vi "BPtrayCalib.vi"(0 "Operation":enum16{"Manual", "Automatic"}(ring)=enum."Automatic", 1 "Zone":enum16{"ZoneA", "ZoneB", "ZoneC", "ZoneD"}(ring), 2 "Autofocus":T4={"Enable"=TRUE, "InitialStepSize"=0.05, "Tolerance"=0.02, "Abort"=FALSE} {"Tolerance" format="%#_13g"}, 7 "StopJoyStick":bool, 9 "VisibilityInCamera":enum16{"JoyStick", "AllVisible"}(ring)=enum."AllVisible", 11 "error in (no error)":errorcluster, 13 "SaveImagesLog":bool=TRUE) -> (6 "Image":T5(plugin-control), 8 "Image 2":T5[](array[plugin-control]) caption="AllImages", 15 "error out":errorcluster)   [LabVIEW 2021]
uses:
  <vilib>/userDefined/High Color/IMAQdx.ctl
  <vilib>/Analysis/coordinate.llb/2D Cartesian Coordinate Rotation (Scalar).vi
  include/GlobalVariables.vi
  Other Models/2010/Motion/AbortSingle.vi
  <vilib>/Analysis/NI_AALPro.lvlib
  <vilib>/vision/driver/NI_Vision_Acquisition_Software.lvlib
panel:
  out "CameraGcode2":string
  out "AllMatches":T1(array[cluster]) {"Bounding Box"."y" format="%.2f"; "Bounding Box"."x" format="%.2f"; "Score" format="%.2f"; "Scale" format="%.2f"; "Angle" format="%.2f"; "Position"."y" format="%.2f"; "Position"."x" format="%.2f"}
  in  "MatchParameters":T2={"Number of Matches Requested"=1, "Minimum Match Score"=500.0, "Angle Ranges"=[{"Start Angle"=0.0, "End Angle"=0.0}]}
  out "OutputFile2":string
  out "XYZU_Back":string
  out "XYZU_Front":string
  out "TrayAngle":dbl
  in  "TrayID":string="1"
  in  "Camera":T3="cam1"
  out "OutputFile1":string
  out "spreadsheet string 2":string
  out "spreadsheet string":string
  in  "ModuleName":string="T1"
  out "SyringeY":dbl format="%#_7g"
  out "SyringeX":dbl format="%#_7g"
  in  "CamToSyringeYoffset":dbl=126.651
  in  "CamToSyringeXoffset":dbl=167.702
  out "FileUsedForFiducials":string
  out "UsedCoordinates":string
  out "CameraGcode1":string
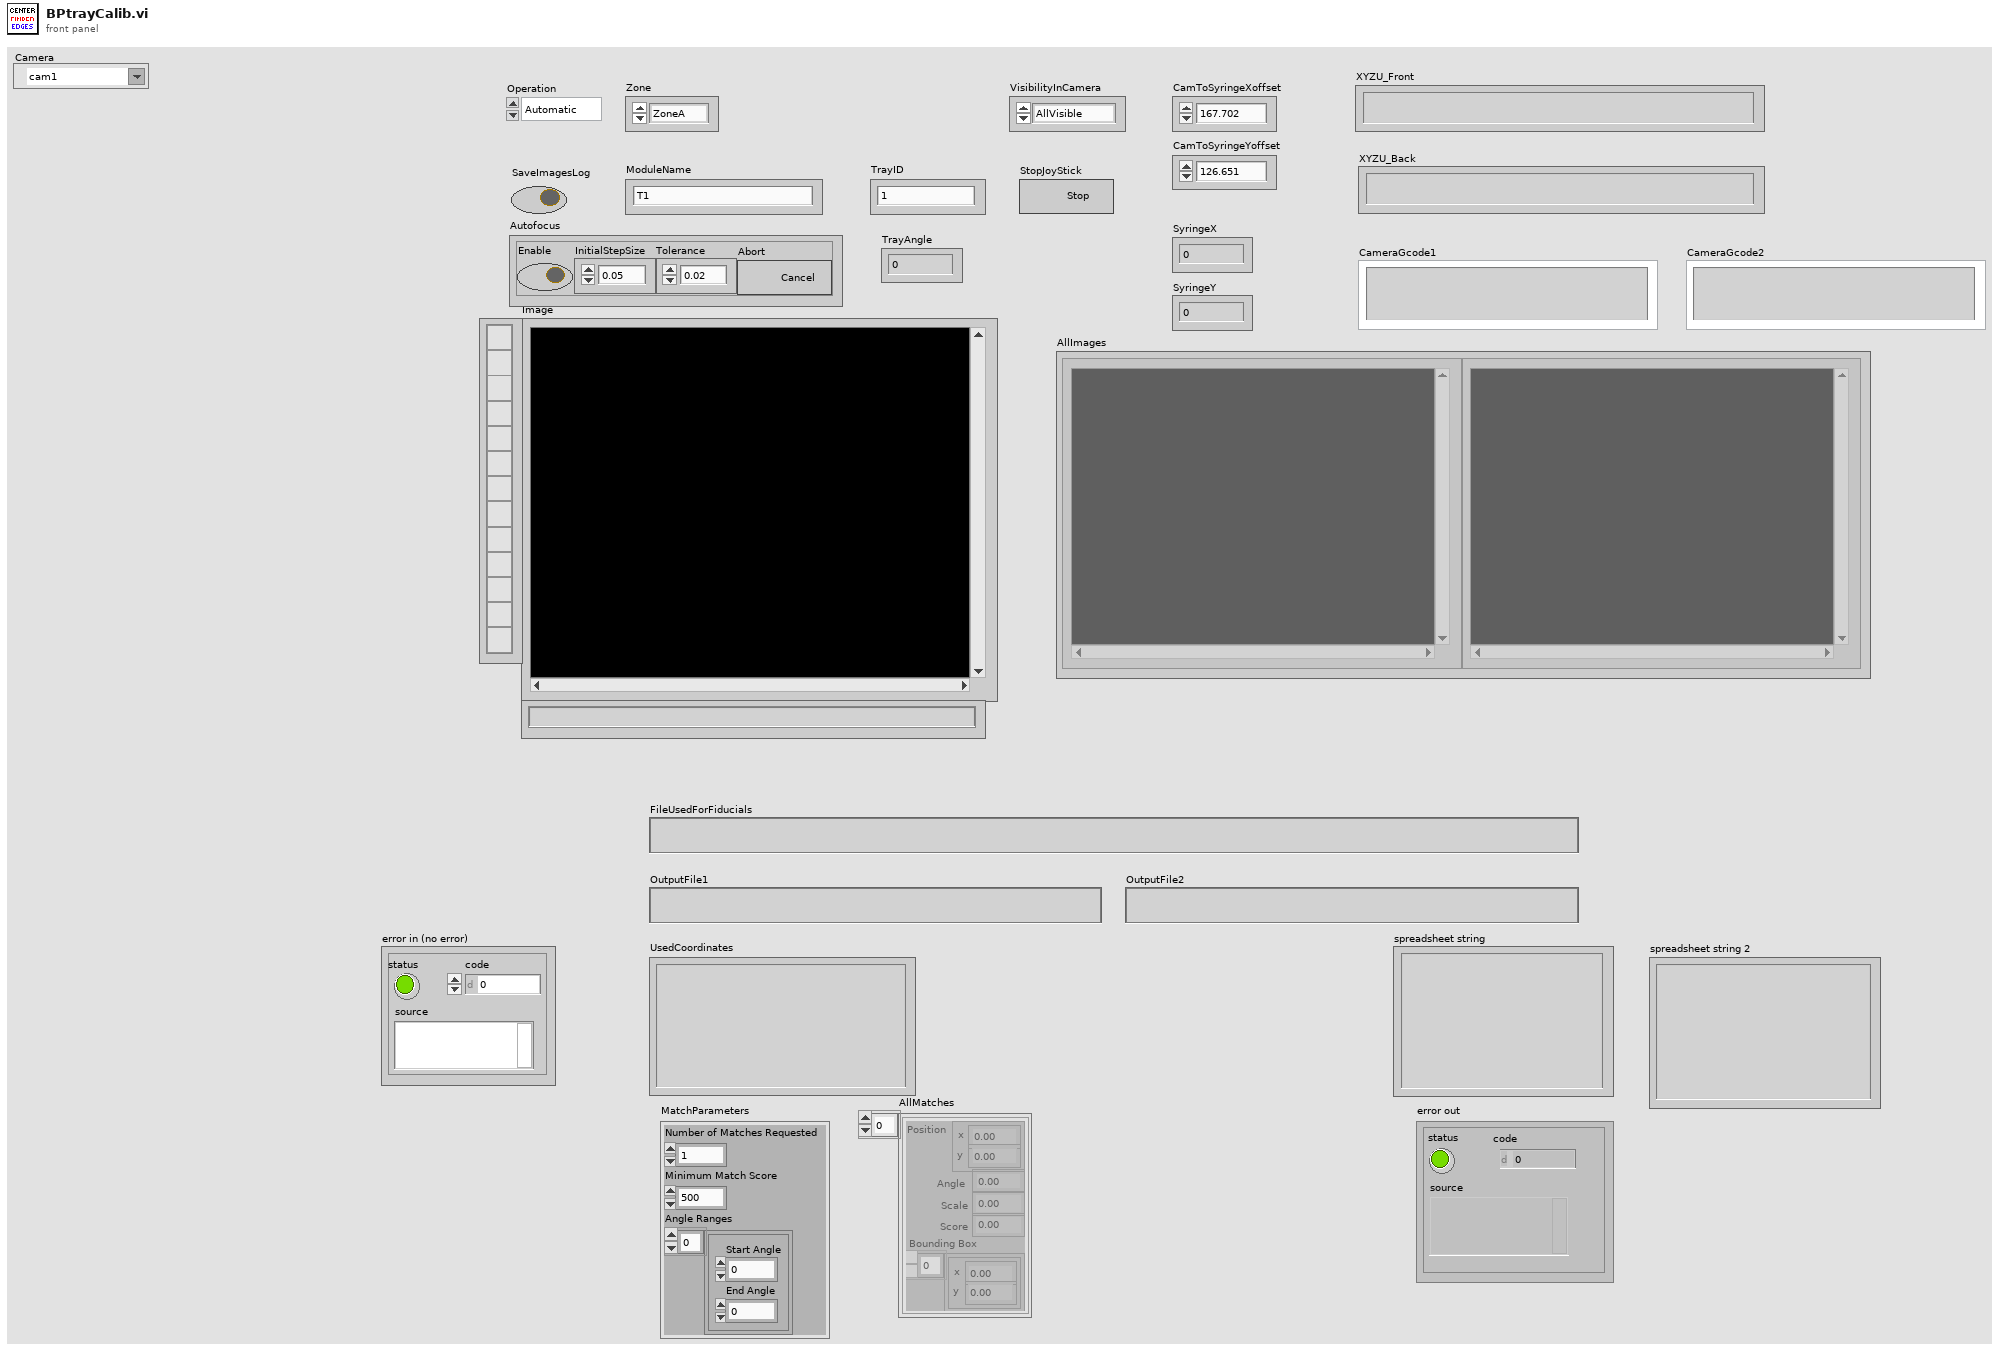
[diagram p1: front panel]
types:
  T1 = cluster{"Position":cluster{"x":sgl, "y":sgl}, "Angle":sgl, "Scale":sgl, "Score":sgl, "Bounding Box":cluster{"x":sgl, "y":sgl}[]}[]
  T2 = cluster{"Number of Matches Requested":i32, "Minimum Match Score":sgl, "Angle Ranges":cluster{"Start Angle":sgl, "End Angle":sgl}[]}
  T3 = typedef "IMAQdx.ctl" = refnum<k21>
  T4 = cluster{"Enable":bool, "InitialStepSize":dbl, "Tolerance":dbl, "Abort":bool}
  T5 = typedef "IMAQ Image.ctl" = refnum<image>
  T6 = typedef "Image Type" = u32
  T7 = typedef "IMAQ Rectangle" = cluster{"Left":i32, "Top":i32, "Right":i32, "Bottom":i32, "Rotation":dbl}
  T8 = enum16{"Left Button", "Center Button", "Right Button", "Window Close"}
  T9 = enum16{"open", "replace", "create", "open or create", "replace or create", "replace or create with confirmation"}
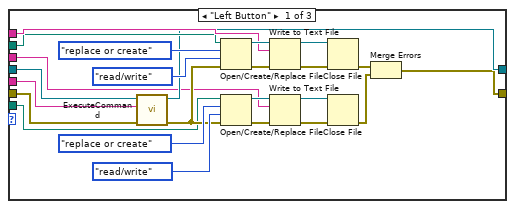
[diagram p3: hidden frame]
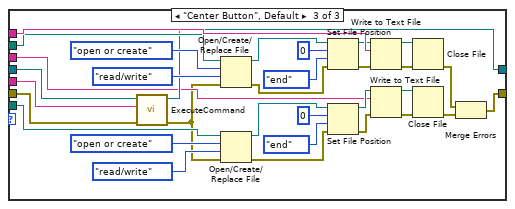
[diagram p4: hidden frame]
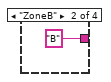
[diagram p5: hidden frame]
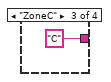
[diagram p6: hidden frame]
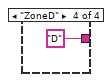
[diagram p7: hidden frame]
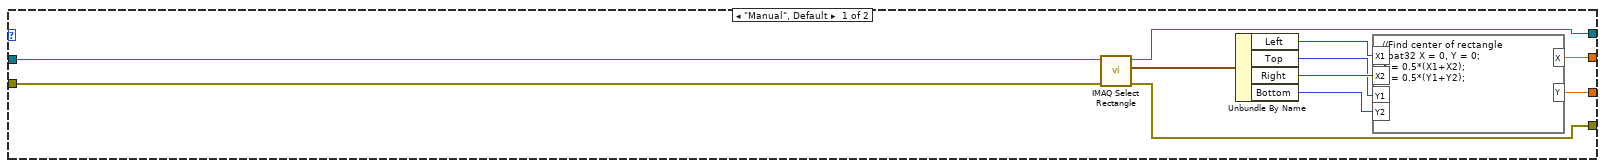
[diagram p8: hidden frame]
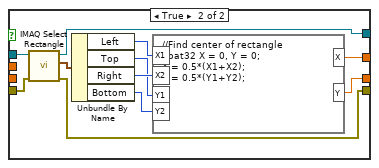
[diagram p9: hidden frame]
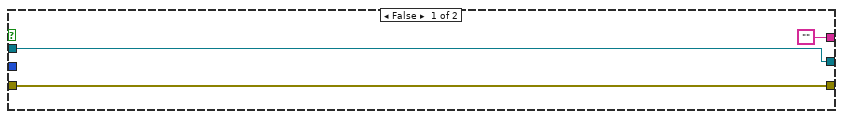
[diagram p10: hidden frame]
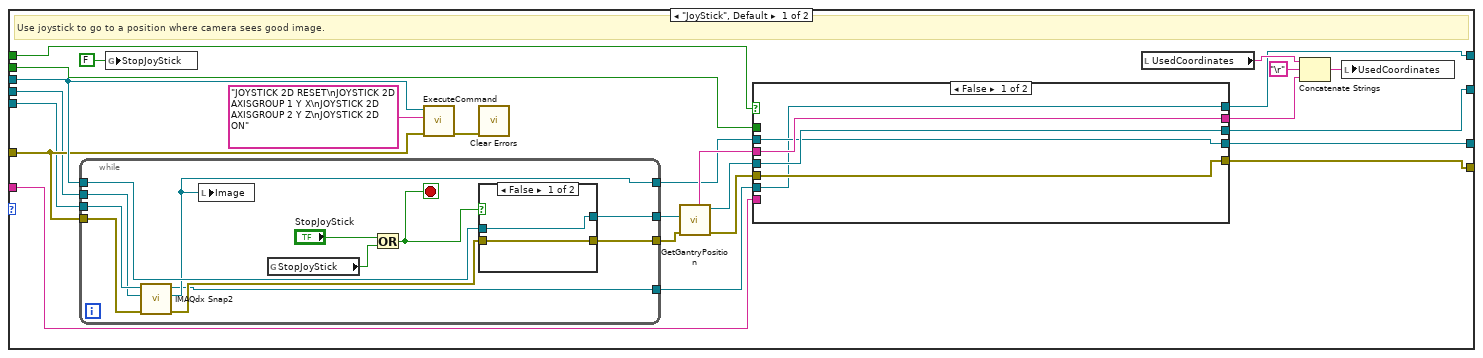
[diagram p11: hidden frame]
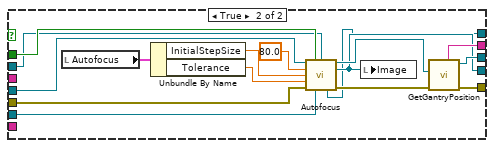
[diagram p12: hidden frame]
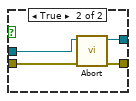
[diagram p13: hidden frame]
diagram:
  w75 = "%f" ("format string")
  w4 = 50.0 ("SpeedZ (mm/s)")
  w5 = 100.0 ("SpeedXY (mm/s)")
  # "Write the XYZU of the baseplate to a text file & move the gantry?"
  # "Prepare to move the gantry to see the center of baseplate in camera."
  # "AllVisble: Assumes that you know the coordinates of all corners (fiducials) well. No need for any adjustments.\nJoyStick: Use joystick at each point to make good image.\nClickMove: Use \"AdjustCamera\" panel and move the gantry stepwise. Click \"Done\" when you're satisfied with the picture."
  n1 = flat-sequence {
    tunnel: [w114] -> w49
    tunnel: [w110] -> w12
    tunnel: [w109] -> w11
    tunnel: [w129] -> w71
    tunnel: [w128] -> w69
    tunnel: w49 -> [w127]
    tunnel: w12 -> [w124]
    tunnel: w11 -> [w123]
    tunnel: w71 -> [w150]
    tunnel: [w150] -> w70
    tunnel: w69 -> [w144]
    tunnel: [w139] -> w68
    tunnel: [w149] -> w67
    tunnel: [w143] -> w60
    tunnel: [w142] -> w59
    tunnel: 2 -> [w176]
    tunnel: "VisibilityInCamera" -> [w169]
    tunnel: w70 -> [w167]
    tunnel: w68 -> [w160]
    tunnel: w67 -> [w166]
    tunnel: w60 -> [w158]
    tunnel: w59 -> [w159]
    tunnel: [w175] -> w58
    tunnel: [w174] -> w57
    tunnel: [w173] -> w56
    tunnel: [w172] -> w55
    tunnel: [w171] -> w54
    tunnel: [w170] -> w53
    tunnel: [w168] -> w52
    tunnel: [w165] -> w51
    tunnel: [w157] -> w50
    tunnel: w58 -> [w443]
    tunnel: w57 -> [w442]
    tunnel: w56 -> [w441]
    tunnel: w55 -> [w440]
    tunnel: w54 -> [w435]
    tunnel: w53 -> [w439]
    tunnel: w52 -> [w438]
    tunnel: w51 -> [w437]
    tunnel: w50 -> [w436]
    tunnel: [w443] -> w48
    tunnel: [w442] -> w46
    tunnel: [w441] -> w44
    tunnel: [w440] -> w42
    tunnel: [w434] -> w40
    tunnel: [w439] -> w38
    tunnel: [w438] -> w36
    tunnel: [w437] -> w34
    tunnel: w48 -> [w453]
    tunnel: [w453] -> w47
    tunnel: w46 -> [w452]
    tunnel: [w452] -> w45
    tunnel: w44 -> [w445]
    tunnel: [w445] -> w43
    tunnel: w42 -> [w460]
    tunnel: [w460] -> w41
    tunnel: w40 -> [w459]
    tunnel: [w459] -> w39
    tunnel: w38 -> [w458]
    tunnel: [w458] -> w37
    tunnel: w36 -> [w457]
    tunnel: [w457] -> w35
    tunnel: w34 -> [w456]
    tunnel: [w456] -> w33
    tunnel: [w449] -> w32
    tunnel: [w448] -> w31
    tunnel: [w447] -> w30
    tunnel: [w444] -> w29
    tunnel: [w538] -> w66
    tunnel: [w539] -> w80
    tunnel: [w540] -> w92
    tunnel: [w517] -> w28
    tunnel: [w541] -> w106
    tunnel: [w542] -> _
    tunnel: [w543] -> w76
    tunnel: [w544] -> w77
    tunnel: w47 -> [w544]
    tunnel: w45 -> [w543]
    tunnel: w43 -> [w542]
    tunnel: w41 -> [w541]
    tunnel: w39 -> [w520]
    tunnel: w37 -> [w540]
    tunnel: w35 -> [w539]
    tunnel: w33 -> [w538]
    tunnel: w32 -> [w515]
    tunnel: w31 -> [w508]
    tunnel: w30 -> [w507]
    tunnel: w29 -> [w501]
    tunnel: [w467] -> w27
    tunnel: [w476] -> w26
    tunnel: [w471] -> w13
    tunnel: [w472] -> w21
    tunnel: [w465] -> w10
    tunnel: [w466] -> w9
    frame #0 {
      w109 = "Configs\\" ("string")
      w110 = "C:\\Users\\TTUHEP\\Documents\\LabVIEW\\GantryPrograms\\"
      w112 = "_BP_Position.txt" ("string")
      n2 = case shown="\"ZoneA\", Default" "Zone" {
        tunnel: ["A" "B" "C" "D"] -> w114
        frame "ZoneA", Default {
        }
        frame "ZoneB" {
        }
        frame "ZoneC" {
        }
        frame "ZoneD" {
        }
      }
      n3 = Concatenate Strings(w110, w109) -> (w108:string)
      n4 = Concatenate Strings(w108, w114, "2", w112) -> (→"OutputFile2":string)
      n5 = Concatenate Strings(w108, w114, "1", w112) -> (→"OutputFile1":string)
      "UsedCoordinates" <- ""
    }
    frame #1 {
      n6 = Concatenate Strings(w124, w123, w127, "_BPtrayFiducials.txt") -> (w125:string)
      "FileUsedForFiducials" <- w125
      n7 = String To Path(string=w125) -> (path=w133:path)
      n8 = Concatenate Strings("This file does not exist:" ("ErrorMessage"), w125) -> (w135:string)
      n9 = call <vilib>:"Check if File or Folder Exists.vi"("error in (no error)"="error in (no error)", "path"=w133) -> ("error out"=w134:errorcluster, "file or folder exists?"=w136:bool, "dup path"=w129:path)  [unwired: 7 in]
      n10 = Not(x=w136) -> (.not. x?=w137:bool)
      n11 = call "AddError.vi"("NoErrorMessage"="InFile OK", "ErrorMessage"=w135, "error in"=w134, "code"=-995, "Error?"=w137) -> ("Error out"=w128:errorcluster)  [unwired: 6 in]
    }
    frame #2 {
      w145 = T6 0 items=["Grayscale (U8)", "Grayscale (I16)", "Grayscale (SGL)", "Complex (CSG)", "RGB (U32)", "HSL (U32)", "RGB (U64)", "Grayscale (U16)"] ("Image Type")
      # "Set the size of the window while selecting the point."
      n12 = call "Connect.vi"("error in (no error)"=w144) -> ("error out"=w152:errorcluster, "controller"=w153:refnum<k24>)  [unwired: 9 in]
      n13 = call "IMAQ WindSize"("Scrollbars? (N)"=TRUE, "Width & Height"=cluster{"Width":i32, "Height":i32} {"Width"=1333, "Height"=1000}, "Window Number"=0) -> ()  [unwired: 3 in, 3 out]
      n14 = call "ExecuteCommand.vi"("error in (no error)"=w152, "Command Code"="G90\nG1 Z0 F100", "controller in"=w153) -> ("error out"=w141:errorcluster, "controller out"=w149:refnum<k24>)  [unwired: 6 in, 1 out]
      n15 = call "IMAQ Create"("Image Name"="name1" ("ImageName"), "Image Type"=w145, "error in (no error)"=w144) -> ("New Image"=w142:T5, "error out"=w147:errorcluster)  [unwired: 2 in]
      n16 = call <vilib>:"IMAQdx Open Camera.vi"("error in"=w147, "Session In"="Camera") -> ("error out"=w140:errorcluster, "Session Out"=w143:T3)  [unwired: 8 in]
      n17 = Merge Errors(w141, w140) -> (w139:errorcluster)
    }
    frame #3 {
      n18 = local read "Autofocus"() -> (w164:T4)
      n19 = local read "Autofocus"() -> (w162:T4)
      n20 = Unbundle By Name(w164) -> ("Enable"=w163:bool)
      n21 = Unbundle By Name(w162) -> ("Abort"=w161:bool)
      n22 = for {
        N: w176 -> [_]
        tunnel: w166 -> [w236]
        tunnel: w167 -> [w219]
        tunnel: [w217] -> w175 mode=indexing
        tunnel: [w216] -> w174 mode=indexing
        tunnel: [w215] -> w173 mode=indexing
        tunnel: [w211] -> w172 mode=indexing
        tunnel: [w210] -> w170
        tunnel: w169 -> [w209]
        tunnel: w161 -> [w208]
        tunnel: w163 -> [w207]
        tunnel: [w203] -> w168
        tunnel: [w198] -> w165 mode=indexing
        shift-right: [w201] -> w171
        shift-left: w160 -> [w185]
        tunnel: w159 -> [w184]
        shift-right: [w178] -> w157
        shift-left: w158 -> [w177]
        i -> [w196]
        w187 = T6 6 items=["Grayscale (U8)", "Grayscale (I16)", "Grayscale (SGL)", "Complex (CSG)", "RGB (U32)", "HSL (U32)", "RGB (U64)", "Grayscale (U16)"] ("Image Type")
        # "Array of XY cluser"
        # "Z array"
        # "Y array"
        # "X array"
        # "Read text file line by line. Each line contains X,Y,Z coordinates for the gantry."
        n23 = call "GetArrayFmTxtFile.vi"("error in"=w185, "LineNo."=w196, "TextFile"=w219) -> ("error out"=w218:errorcluster, "Array"=w243:dbl[])
        n24 = Index Array(array=w243, index=0) -> (element=w238:dbl)
        n25 = Index Array(array=w243, index=1) -> (element=w237:dbl)
        n26 = Index Array(array=w243, index=2) -> (element=w239:dbl)
        n27 = call "Move.vi"("X"=w238, "Absolute"=TRUE, "Y"=w237, "Z"=w239, "SpeedXY (mm/s)"=100.0, "SpeedZ (mm/s)"=100.0, "Move Z first"=FALSE) -> ("Position Gcode"=w235:string)  [unwired: 8 in]
        n28 = call "ExecuteCommand.vi"("error in (no error)"=w218, "Command Code"=w235, "controller in"=w236) -> ("error out"=w183:errorcluster, "controller out"=w234:refnum<k24>)  [unwired: 6 in, 1 out]
        n29 = call <vilib>:"IMAQdx Snap2.vi"("error in"=w183, "Image In"=w184, "Session In"=w177) -> ("error out"=w182:errorcluster, "Image Out"=w180:T5, "Session Out"=w181:T3)  [unwired: 6 in]
        n30 = local write "Image"(w180) -> ()
        n31 = case shown="\"AllVisible\"" w209 {
          tunnel: w181 -> [w341 w403]
          tunnel: w234 -> [w359 w415]
          tunnel: w182 -> [w357 w416]
          tunnel: [w337 w404] -> w205
          tunnel: [w346 w410] -> w223
          tunnel: [w347 w408] -> w179
          tunnel: w208 -> [w350 w413]
          tunnel: w207 -> [w344 w414]
          tunnel: "name1" ("ImageName") -> [w343 w402]
          tunnel: w180 -> [w340 w401]
          tunnel: [w336 w400] -> w178
          frame "JoyStick", Default {
            # "Use joystick to go to a position where camera sees good image."
            n32 = while {
              tunnel: [w387] -> w338
              tunnel: w359 -> [w393]
              tunnel: [w392] -> w355
              tunnel: [w391] -> w356
              tunnel: w357 -> [w386]
              tunnel: w341 -> [w384]
              tunnel: w340 -> [w383]
              tunnel: [w382] -> w339
              stop <- w388 stop-if-true
              n33 = call <vilib>:"IMAQdx Snap2.vi"("error in"=w386, "Image In"=w383, "Session In"=w384) -> ("error out"=w385:errorcluster, "Image Out"=w387:T5, "Session Out"=w382:T3)  [unwired: 6 in]
              n34 = local write "Image"(w387) -> ()
              n35 = global read "GlobalVariables.vi" "StopJoyStick"() -> (w389:bool)
              n36 = Or(x="StopJoyStick", y=w389) -> (x .or. y?=w388:bool)
              n37 = case shown="False" w388 {
                tunnel: w393 -> [w395 w399]
                tunnel: w385 -> [w394 w398]
                tunnel: [w394 w397] -> w392
                tunnel: [w395 w396] -> w391
                frame False {
                }
                frame True {
                  n38 = call-poly "Abort.vi"("error in (no error)"=w398, "controller in"=w399) -> ("error out"=w397:errorcluster, "controller out"=w396:refnum<k24>)  [unwired: 8 in]
                }
              }
            }
            n39 = global write "GlobalVariables.vi" "StopJoyStick"(FALSE ("StopJoyStick")) -> ()
            n40 = call "ExecuteCommand.vi"("error in (no error)"=w357, "Command Code"="JOYSTICK 2D RESET\nJOYSTICK 2D AXISGROUP 1 Y X\nJOYSTICK 2D AXISGROUP 2 Y Z\nJOYSTICK 2D ON", "controller in"=w359) -> ("error out"=w358:errorcluster)  [unwired: 6 in, 2 out]
            n41 = call <vilib>:"Clear Errors.vi"("error in (no error)"=w358) -> ()  [unwired: 5 in, 2 out]
            n42 = call "GetGantryPosition.vi"("error in (no error)"=w355, "Controller In"=w356) -> ("error out"=w351:errorcluster, "controller out"=w349:refnum<k24>, "Position_XYZ"=w345:string)  [unwired: 3 in, 4 out]
            n43 = case shown="False" w344 {
              tunnel: w351 -> [w365 w381]
              tunnel: w350 -> [_ w374]
              tunnel: w349 -> [w363 w375]
              tunnel: [w364 w379] -> w348
              tunnel: [w365 w378] -> w347
              tunnel: [w363 w377] -> w346
              tunnel: w345 -> [w364 _]
              tunnel: w343 -> [_ _]
              tunnel: w339 -> [w361 w369]
              tunnel: w338 -> [w362 w368]
              tunnel: [w362 w367] -> w337
              tunnel: [w361 w366] -> w336
              frame False {
              }
              frame True {
                n44 = local read "Autofocus"() -> (w372:T4)
                n45 = Unbundle By Name(w372) -> ("InitialStepSize"=w370:dbl, "Tolerance"=w371:dbl)
                n46 = call "Autofocus.vi"("controller in"=w375, "AbortAutoFocus"=w374, "ImageIn"=w368, "SafeMaxZ"=80.0, "InitialStepSize"=w370, "Tolerance"=w371, "error in (no error)"=w381, "SessionIn"=w369) -> ("controller out"=w380:refnum<k24>, "Image"=w367:T5, "Session Out"=w366:T3, "error out"=w376:errorcluster)  [unwired: 2 in, 2 out]
                n47 = local write "Image"(w367) -> ()
                n48 = call "GetGantryPosition.vi"("error in (no error)"=w376, "Controller In"=w380) -> ("error out"=w378:errorcluster, "controller out"=w377:refnum<k24>, "Position_XYZ"=w379:string)  [unwired: 3 in, 4 out]
              }
            }
            n49 = local read "UsedCoordinates"() -> (w353:string)
            n50 = Concatenate Strings(w353, "\r", w348) -> (w354:string)
            n51 = local write "UsedCoordinates"(w354) -> ()
          }
          frame "AllVisible" {
            # "No need to move gantry to take a good pic."
            n52 = case shown="True" w414 {
              tunnel: w413 -> [_ w428]
              tunnel: [w420 w431] -> w409
              tunnel: [w419 w433] -> w411
              tunnel: w416 -> [w420 w432]
              tunnel: w415 -> [w419 w430]
              tunnel: [w418 w427] -> w404
              tunnel: w403 -> [w417 w423]
              tunnel: w402 -> [_ _]
              tunnel: w401 -> [w418 w422]
              tunnel: [w417 w421] -> w400
              frame False {
              }
              frame True {
                n53 = local read "Autofocus"() -> (w426:T4)
                n54 = Unbundle By Name(w426) -> ("InitialStepSize"=w425:dbl, "Tolerance"=w424:dbl)
                n55 = call "Autofocus.vi"("controller in"=w430, "AbortAutoFocus"=w428, "ImageIn"=w422, "SafeMaxZ"=84.0, "InitialStepSize"=w425, "Tolerance"=w424, "error in (no error)"=w432, "SessionIn"=w423) -> ("controller out"=w433:refnum<k24>, "Image"=w427:T5, "Session Out"=w421:T3, "error out"=w431:errorcluster)  [unwired: 2 in, 2 out]
                n56 = local write "Image"(w427) -> ()
              }
            }
            n57 = local read "UsedCoordinates"() -> (w406:string)
            n58 = call "GetGantryPosition.vi"("error in (no error)"=w409, "Controller In"=w411) -> ("error out"=w408:errorcluster, "controller out"=w410:refnum<k24>, "Position_XYZ"=w407:string)  [unwired: 3 in, 4 out]
            n59 = Concatenate Strings(w406, "\r", w407) -> (w405:string)
            n60 = local write "UsedCoordinates"(w405) -> ()
          }
        }
        n61 = case shown="\"Automatic\"" "Operation" {
          tunnel: [w252 w267] -> w231
          tunnel: [w251 w266] -> w230
          tunnel: [w247 w275] -> w229
          tunnel: w179 -> [w249 w289]
          tunnel: w205 -> [w250 w292]
          tunnel: [w248 w273] -> w197
          frame "Manual", Default {
            n62 = call "IMAQ Select Rectangle"("error in (no error)"=w249, "Image In"=w250) -> ("error out"=w247:errorcluster, "Rectangle"=w257:T7, "Image Out (duplicate)"=w248:T5)  [unwired: 6 in, 1 out]
            n63 = Unbundle By Name(w257) -> ("Left"=w256:i32, "Top"=w254:i32, "Right"=w255:i32, "Bottom"=w253:i32)
            n64 = formula code="//Find center of rectangle\nfloat32 X = 0, Y = 0;\nX = 0.5*(X1+X2);\nY = 0.5*(Y1+Y2);"("X1"=w256, "X2"=w255, "Y1"=w254, "Y2"=w253) -> ("X"=w252:sgl, "Y"=w251:sgl)
          }
          frame "Automatic" {
            w260 = "TLM_Circle"
            w271 = sgl 50.0 ("y")
            w287 = ""
            n65 = Concatenate Strings("Could not parse/find this template file for pattern recognition:" ("ErrorMessage"), w260) -> (w282:string)
            n66 = call "JSONfileReader.vi"("error in"=w289, "Variant"=w287, "ItemName"=w260, "FileIn"=path "C:/Users/TTUHEP/Documents/LabVIEW/GantryPrograms/Configs/PatternRecognTemplateMaps.json" ("PatterRecognTemplateMap")) -> ("error out"=w279:errorcluster, "Data"=w288:variant, "Found"=w285:bool)
            n67 = Not(x=w285) -> (.not. x?=w284:bool)
            n68 = Variant To Data(error in=w279, type=w287, Variant=w288) -> (data=w286:string, error out=w278:errorcluster)
            n69 = call "AddError.vi"("NoErrorMessage"="Template file name found from json.", "ErrorMessage"=w282, "error in"=w278, "code"=-902, "Error?"=w284) -> ("Error out"=w277:errorcluster)  [unwired: 6 in]
            n70 = call "PatternRecognition.vi"("error in (no error)"=w277, "MatchParameters"="MatchParameters", "ImageIn"=w292, "TemplateFileName"=w286) -> ("error out"=w262:errorcluster, "AllMatches"=→"AllMatches":T1, "Position"=w291:cluster{"x":sgl, "y":sgl}, "ImageFoundPattern"=w274:T5, "Number of Matches"=w276:i32)  [unwired: 2 in]
            n71 = Equal To 0?(x=w276) -> (x = 0?=w272:bool)
            n72 = Unbundle(w291) -> ("x"=w265:sgl, "y"=w264:sgl)
            n73 = call <vilib>:"Clear Errors.vi"("error in (no error)"=w262, "specific error code to clear (0: all)"=-903) -> ("error out"=w261:errorcluster)  [unwired: 4 in, 1 out]
            n74 = Less?(x=w265, y=w271) -> (x < y?=w270:bool)
            n75 = Less?(x=w264, y=w271) -> (x < y?=w269:bool)
            n76 = Compound Arithmetic op=OR(w272, w270, w269) -> (w268:bool)
            n77 = case shown="False" w268 {
              tunnel: w261 -> [w296 w302]
              tunnel: [w296 w299] -> w275
              tunnel: w274 -> [w295 w297]
              tunnel: [w295 w298] -> w273
              tunnel: [w294 w301] -> w267
              tunnel: [w293 w300] -> w266
              tunnel: w265 -> [w294 _]
              tunnel: w264 -> [w293 _]
              frame False {
              }
              frame True {
                n78 = call "IMAQ Select Rectangle"("error in (no error)"=w302, "Image In"=w297) -> ("error out"=w299:errorcluster, "Rectangle"=w307:T7, "Image Out (duplicate)"=w298:T5)  [unwired: 6 in, 1 out]
                n79 = Unbundle By Name(w307) -> ("Left"=w306:i32, "Top"=w304:i32, "Right"=w305:i32, "Bottom"=w303:i32)
                n80 = formula code="//Find center of rectangle\nfloat32 X = 0, Y = 0;\nX = 0.5*(X1+X2);\nY = 0.5*(Y1+Y2);"("X1"=w306, "X2"=w305, "Y1"=w304, "Y2"=w303) -> ("X"=w301:sgl, "Y"=w300:sgl)
              }
            }
          }
        }
        n81 = Number To Decimal String(number=w196) -> (decimal integer string=w195:string)  [unwired: 1 in]
        n82 = Concatenate Strings("imgTemp" ("string"), w195) -> (w192:string)
        n83 = call "GetPixelToGantryRelPosition.vi"("error in (no error)"=w229, "PixelY"=w230, "PixelX"=w231) -> ("error out"=w190:errorcluster, "YmmRelGH"=w227:dbl, "XmmRelGH"=w228:dbl)
        n84 = call "IMAQ Create"("Image Name"=w192, "Image Type"=w187, "error in (no error)"=w190) -> ("New Image"=w191:T5, "error out"=w189:errorcluster)  [unwired: 2 in]
        n85 = call "IMAQ Copy"("error in (no error)"=w189, "Image Dst"=w191, "Image Src"=w197) -> ("error out"=w188:errorcluster, "Image Dst Out"=w193:T5)  [unwired: 3 in]
        n86 = Build Array(w193) -> (w198:T5[])
        n87 = flat-sequence {
          tunnel: w188 -> [w327]
          tunnel: [w327] -> w233
          tunnel: w223 -> [w326]
          tunnel: [w326] -> w232
          tunnel: [w335] -> w202
          tunnel: [w334] -> w226
          tunnel: [w333] -> w225
          tunnel: [w332] -> w210
          tunnel: [w331] -> w224
          tunnel: w233 -> [w330]
          tunnel: w232 -> [w329]
          frame #0 {
            n88 = Wait (ms)(milliseconds to wait=u32 1000) -> ()  [unwired: 1 out]
          }
          frame #1 {
            n89 = call "GetGantryPosition.vi"("error in (no error)"=w330, "Controller In"=w329) -> ("error out"=w335:errorcluster, "Position Y"=w334:dbl, "Position X"=w333:dbl, "controller out"=w332:refnum<k24>, "Position Z"=w331:dbl)  [unwired: 3 in, 2 out]
          }
        }
        n90 = Add(x=w228, y=w225) -> (x+y=w222:dbl)
        n91 = Add(x=w227, y=w226) -> (x+y=w221:dbl)
        n92 = case shown="True" "SaveImagesLog" {
          tunnel: w197 -> [w308 w325]
          tunnel: w196 -> [_ w323]
          tunnel: ["" w315] -> w203
          tunnel: w202 -> [w309 w314]
          tunnel: [w309 w313] -> w201
          tunnel: [w308 w312] -> w186
          frame False {
          }
          frame True {
            w317 = "C:\\Users\\TTUHEP\\Documents\\LabVIEW\\GantryPrograms\\LogFiles\\CalibrationData\\"
            n93 = Number To Decimal String(number=w323) -> (decimal integer string=w321:string)  [unwired: 1 in]
            n94 = Concatenate Strings(w317, "ModuleName") -> (w315:string)
            n95 = Concatenate Strings(w317, "ModuleName", "TLMfid", "Image" ("string"), w321, ".png" ("string")) -> (w319:string)
            n96 = String To Path(string=w319) -> (path=w318:path)
            n97 = call-poly "IMAQ Write File 2"("error in (no error)"=w314, "Image Quality"=u32 1000, "File Path"=w318, "Image"=w325) -> ("error out"=w313:errorcluster, "Image Out (duplicate)"=w312:T5)  [unwired: 6 in]
          }
        }
        "Image" <- w186
        n98 = call-poly <vilib>:"2D Cartesian Coordinate Rotation.vi"("theta"=0.0, "y"=w221, "x"=w222) -> ("y out"=w213:dbl, "x out"=w214:dbl)  [unwired: 6 in, 1 out]
        n99 = global write "GlobalVariables.vi" "Image"(w186) -> ()
        n100 = Bundle("x out"=w214, "y out"=w213) -> (w212:cluster{"x out":dbl, "y out":dbl})  [unwired: 1 in]
        n101 = Build Array(w212) -> (w211:cluster{"x out":dbl, "y out":dbl}[])
        n102 = Build Array(w214) -> (w217:dbl[])
        n103 = Build Array(w213) -> (w216:dbl[])
        n104 = Build Array(w224) -> (w215:dbl[])
      }
    }
    frame #4 {
      n105 = call <vilib>:"IMAQdx Close Camera.vi"("error in"=w435, "Session In"=w436) -> ("error out"=w434:errorcluster)  [unwired: 9 in]
    }
    frame #5 {
      n106 = Index Array "X"(array=w453, index (col)=0 ("disabled index (col)")) -> (element=w451:dbl[])  [unwired: 1 in]
      n107 = Index Array "Y"(array=w452, index (col)=0 ("disabled index (col)")) -> (element=w450:dbl[])  [unwired: 1 in]
      n108 = Index Array "Z"(array=w445, index (col)=0) -> (element=w444:dbl[])  [unwired: 1 in]
      n109 = formula code="float64 angl_r = (yin[0] - yin[1]) / (xin[0] - xin[1]);\nfloat64 angl = (atan(angl_r)*180.0/3.14159);\nfloat64 FidMidX = 0.5*(xin[0]+xin[1]);\nfloat64 FidMidY = 0.5*(yin[0]+yin[1]);"("xin"=w451, "yin"=w450) -> ("angl"=w449:dbl, "FidMidX"=w448:dbl, "FidMidY"=w447:dbl)
      "TrayAngle" <- w449
    }
    frame #6 {
      w473 = "\r"
      w486 = "\t"
      w488 = "\t"
      # "Calc rotation of slotPinLine"
      # "Calc rotation of slotPinLine"
      n110 = Index Array(array=w501, index=0) -> (element=w500:dbl)
      n111 = Index Array(array=w501, index=1) -> (element=w498:dbl)
      n112 = Concatenate Strings("C:\\Users\\TTUHEP\\Documents\\LabVIEW\\GantryPrograms\\Configs\\TrayID" ("string"), "TrayID", "_FiducialsPins.txt") -> (w534:string)
      n113 = String To Path(string=w534) -> (path=w519:path)
      n114 = call "GetArrayFmTxtFile.vi"("error in"=w520, "LineNo."=0, "TextFile"=w519) -> ("error out"=w518:errorcluster, "Array"=w529:dbl[])
      n115 = call "GetArrayFmTxtFile.vi"("error in"=w520, "LineNo."=1, "TextFile"=w519) -> ("error out"=w516:errorcluster, "Array"=w523:dbl[])
      n116 = Merge Errors(w518, w516) -> (w517:errorcluster)
      n117 = Index Array(array=w529, index=0) -> (element=w514:dbl)
      n118 = Index Array(array=w529, index=1) -> (element=w513:dbl)
      n119 = Index Array(array=w529, index=3) -> (element=w470:dbl)
      n120 = Index Array(array=w529, index=2) -> (element=w504:dbl)
      n121 = Index Array(array=w523, index=0) -> (element=w512:dbl)
      n122 = Index Array(array=w523, index=1) -> (element=w511:dbl)
      n123 = Index Array(array=w523, index=3) -> (element=w522:dbl)
      n124 = Index Array(array=w523, index=2) -> (element=w499:dbl)
      n125 = Add(x=w515, y=w470) -> (x+y=w468:dbl)
      n126 = Add(x=w504, y=w500) -> (x+y=w471:dbl)
      n127 = Add(x=w515, y=w522) -> (x+y=w469:dbl)
      n128 = Add(x=w499, y=w498) -> (x+y=w489:dbl)
      n129 = expression code="(x/180.0)*pi" "degrees to radians"(w468) -> (w462:dbl)
      n130 = expression code="(x/180.0)*pi" "degrees to radians"(w469) -> (w464:dbl)
      n131 = Negate(x=w462) -> (-x=w461:dbl)
      n132 = Negate(x=w464) -> (-x=w463:dbl)
      n133 = call-poly <vilib>:"2D Cartesian Coordinate Rotation.vi"("theta"=w461, "y"=w513, "x"=w514) -> ("y out"=w509:dbl, "x out"=w510:dbl)  [unwired: 6 in, 1 out]
      n134 = call-poly <vilib>:"2D Cartesian Coordinate Rotation.vi"("theta"=w463, "y"=w511, "x"=w512) -> ("y out"=w506:dbl, "x out"=w505:dbl)  [unwired: 6 in, 1 out]
      n135 = Add(x=w510, y=w508) -> (x+y=w467:dbl)
      n136 = Add(x=w509, y=w507) -> (x+y=w476:dbl)
      n137 = Add(x=w508, y=w505) -> (x+y=w465:dbl)
      n138 = Add(x=w507, y=w506) -> (x+y=w466:dbl)
      n139 = Number To Fractional String(number=w467, precision (6)=i16 4 ("width (-)")) -> (F-format string=w484:string)  [unwired: 2 in]
      n140 = Number To Fractional String(number=w476, precision (6)=i16 4 ("width (-)")) -> (F-format string=w483:string)  [unwired: 2 in]
      n141 = Number To Fractional String(number=w471, precision (6)=i16 4 ("width (-)")) -> (F-format string=w482:string)  [unwired: 2 in]
      n142 = Number To Fractional String(number=w468, precision (6)=i16 4 ("width (-)")) -> (F-format string=w481:string)  [unwired: 2 in]
      n143 = Number To Fractional String(number=w465, precision (6)=i16 4 ("width (-)")) -> (F-format string=w480:string)  [unwired: 2 in]
      n144 = Number To Fractional String(number=w466, precision (6)=i16 4 ("width (-)")) -> (F-format string=w479:string)  [unwired: 2 in]
      n145 = Number To Fractional String(number=w489, precision (6)=i16 4 ("width (-)")) -> (F-format string=w478:string)  [unwired: 2 in]
      n146 = Number To Fractional String(number=w469, precision (6)=i16 4 ("width (-)")) -> (F-format string=w477:string)  [unwired: 2 in]
      n147 = Concatenate Strings(w484, w488, w483, w488, w482, w488, w481, "\r") -> (w475:string)
      "XYZU_Front" <- w475
      n148 = Concatenate Strings(w480, w486, w479, w486, w478, w486, w477, "\r") -> (w474:string)
      "XYZU_Back" <- w474
      n149 = Concatenate Strings(w473, w475, w473, w474, w473) -> (w472:string)
    }
  }
  n150 = Array To Spreadsheet String(array=w76, 3:w75) -> (spreadsheet string=→"spreadsheet string 2":string)  [unwired: 1 in]
  n151 = Array To Spreadsheet String(array=w77, 3:w75) -> (spreadsheet string=→"spreadsheet string":string)  [unwired: 1 in]
  n152 = local read "OutputFile1"() -> (w25:string)
  n153 = local read "OutputFile2"() -> (w23:string)
  n154 = call "CameraXYusingGantryHeadXY.vi"("GantryY"=w9, "GantryX"=w10) -> ("CamY"=w7:dbl, "CamX"=w8:dbl)
  n155 = call "CameraXYusingGantryHeadXY.vi"("GantryY"=w26, "GantryX"=w27) -> ("CamY"=w86:dbl, "CamX"=w88:dbl)
  n156 = Index Array(array=w66, index (col)=0 ("disabled index (col)")) -> (element=→"Image 2":T5[])  [unwired: 1 in]
  n157 = Greater?(x=w13, y=83.0) -> (0:w15:bool)
  n158 = Index Array "Points"(array=w106, index (col)=0 ("disabled index (col)")) -> ()  [unwired: 1 in, 1 out]
  n159 = Concatenate Strings("Overwrite/Append ", w21, " to files ", w25, " and " ("string"), w23, " ?" ("string")) -> (w101:string)
  n160 = Select(t=0.0, s=w15, f=w13) -> (s? t:f=w6:dbl)
  n161 = Add(x="CamToSyringeYoffset", y=w86) -> (x+y=→"SyringeY":dbl)
  n162 = local read "OutputFile1"() -> (w18:string)
  n163 = local read "OutputFile2"() -> (w17:string)
  n164 = call "Move.vi"("X"=w8, "Absolute"=TRUE, "Y"=w7, "Z"=w6, "SpeedXY (mm/s)"=w5, "SpeedZ (mm/s)"=w4, "Move Z first"=TRUE) -> ("Position Gcode"=→"CameraGcode2":string)  [unwired: 8 in]
  n165 = call "Move.vi"("X"=w88, "Absolute"=TRUE, "Y"=w86, "Z"=w6, "SpeedXY (mm/s)"=w5, "SpeedZ (mm/s)"=w4, "Move Z first"=TRUE) -> ("Position Gcode"=w95:string)  [unwired: 8 in]
  "CameraGcode1" <- w95
  n166 = call <vilib>:"Three Button Dialog.vi"("Right Button Text (\"Cancel\")"="Do nothing" ("Right Button Text (\"Cancel\")"), "Center Button Text (\"No\")"="Append" ("Center Button Text (\"No\")"), "Left Button Text (\"Yes\")"="Overwrite" ("Left Button Text (\"Yes\")"), "message"=w101) -> ("Which Button?"=w100:T8)  [unwired: 7 in]
  n167 = Add(x="CamToSyringeXoffset", y=w88) -> (x+y=→"SyringeX":dbl)
  n168 = String To Path(string=w18) -> (path=w72:path)
  n169 = String To Path(string=w17) -> (path=w22:path)
  n170 = local read "XYZU_Front"() -> (w20:string)
  n171 = local read "XYZU_Back"() -> (w19:string)
  n172 = case shown="\"Right Button\"" w100 {
    tunnel: w20 -> [w562 _ w598]
    tunnel: w72 -> [w561 _ w597]
    tunnel: w28 -> [w560 w570 w596]
    tunnel: w95 -> [w559 _ w595]
    tunnel: w92 -> [w558 w569 w594]
    tunnel: [w545 w570 w572] -> w82
    tunnel: [w557 w569 w593] -> w94
    tunnel: w22 -> [w549 _ w575]
    tunnel: w19 -> [w548 _ w576]
    frame "Left Button" {
      n173 = call "ExecuteCommand.vi"("error in (no error)"=w560, "Command Code"=w559, "controller in"=w558) -> ("error out"=w550:errorcluster, "controller out"=w557:refnum<k24>)  [unwired: 6 in, 1 out]
      n174 = Open/Create/Replace File(file path (use dialog)=w561, error in=w550, operation (0:open)=T9."replace or create", access (0:read/write)=enum16{"read/write", "read-only", "write-only"}."read/write") -> (refnum out=w568:refnum<file>, error out=w565:errorcluster)  [unwired: 2 in, 1 out]
      n175 = Open/Create/Replace File(file path (use dialog)=w549, error in=w550, operation (0:open)=T9."replace or create", access (0:read/write)=enum16{"read/write", "read-only", "write-only"}."read/write") -> (refnum out=w556:refnum<file>, error out=w553:errorcluster)  [unwired: 2 in, 1 out]
      n176 = Write to Text File(file (use dialog)=w568, text=w562, error in=w565) -> (refnum out=w563:refnum<file>, error out=w564:errorcluster)  [unwired: 1 in, 1 out]
      n177 = Write to Text File(file (use dialog)=w556, text=w548, error in=w553) -> (refnum out=w551:refnum<file>, error out=w552:errorcluster)  [unwired: 1 in, 1 out]
      n178 = Close File(refnum=w563, error in=w564) -> (error out=w547:errorcluster)  [unwired: 1 out]
      n179 = Close File(refnum=w551, error in=w552) -> (error out=w546:errorcluster)  [unwired: 1 out]
      n180 = Merge Errors(w547, w546) -> (w545:errorcluster)
    }
    frame "Right Button" {
    }
    frame "Center Button", Default {
      n181 = call "ExecuteCommand.vi"("error in (no error)"=w596, "Command Code"=w595, "controller in"=w594) -> ("error out"=w574:errorcluster, "controller out"=w593:refnum<k24>)  [unwired: 6 in, 1 out]
      n182 = Open/Create/Replace File(file path (use dialog)=w597, error in=w574, operation (0:open)=T9."open or create", access (0:read/write)=enum16{"read/write", "read-only", "write-only"}."read/write") -> (refnum out=w590:refnum<file>, error out=w588:errorcluster)  [unwired: 2 in, 1 out]
      n183 = Open/Create/Replace File(file path (use dialog)=w575, error in=w574, operation (0:open)=T9."open or create", access (0:read/write)=enum16{"read/write", "read-only", "write-only"}."read/write") -> (refnum out=w580:refnum<file>, error out=w578:errorcluster)  [unwired: 2 in, 1 out]
      n184 = Set File Position(offset (in bytes) (0)=i64 0, refnum=w590, from (0:start)=enum16{"start", "end", "current"}."end", error in=w588) -> (refnum out=w589:refnum<file>, error out=w587:errorcluster)
      n185 = Set File Position(offset (in bytes) (0)=i64 0, refnum=w580, from (0:start)=enum16{"start", "end", "current"}."end", error in=w578) -> (refnum out=w579:refnum<file>, error out=w577:errorcluster)
      n186 = Write to Text File(file (use dialog)=w589, text=w598, error in=w587) -> (refnum out=w599:refnum<file>, error out=w600:errorcluster)  [unwired: 1 in, 1 out]
      n187 = Write to Text File(file (use dialog)=w579, text=w576, error in=w577) -> (refnum out=w583:refnum<file>, error out=w584:errorcluster)  [unwired: 1 in, 1 out]
      n188 = Close File(refnum=w599, error in=w600) -> (error out=w573:errorcluster)  [unwired: 1 out]
      n189 = Close File(refnum=w583, error in=w584) -> (error out=w571:errorcluster)  [unwired: 1 out]
      n190 = Merge Errors(w573, w571) -> (w572:errorcluster)
    }
  }
  n191 = call "CaptureImage.vi"("Camera"=T3 "cam1", "ImageName"="CurrImage", "Draw50MicroCircleAtCenter"=TRUE, "error in (no error)"=w82) -> ("Image"=w63:T5, "error out"=w81:errorcluster)  [unwired: 3 in]
  n192 = local write "Image"(w63) -> ()
  n193 = global write "GlobalVariables.vi" "Image"(w63) -> ()
  n194 = call "Disconnect.vi"("error in (no error)"=w81, "controller"=w94) -> ("error out"=w78:errorcluster)  [unwired: 9 in]
  n195 = local read "SaveImagesLog"() -> (w83:bool)
  n196 = case shown="True" w83 {
    tunnel: w78 -> [w603 w618]
    tunnel: w80 -> [_ w611]
    tunnel: w63 -> [_ w606]
    tunnel: [w603 w604] -> w79
    frame False {
    }
    frame True {
      n197 = Concatenate Strings(w611, "UsedXYZ.txt") -> (w616:string)
      n198 = local read "UsedCoordinates"() -> (w613:string)
      n199 = Concatenate Strings(w611, "CenterImage.png") -> (w609:string)
      n200 = String To Path(string=w616) -> (path=w615:path)
      n201 = String To Path(string=w609) -> (path=w607:path)
      n202 = Open/Create/Replace File(file path (use dialog)=w615, error in=w618, operation (0:open)=T9."open or create", access (0:read/write)=enum16{"read/write", "read-only", "write-only"}."read/write") -> (refnum out=w614:refnum<file>, error out=w622:errorcluster)  [unwired: 2 in, 1 out]
      n203 = Write to Text File(file (use dialog)=w614, text=w613, error in=w622) -> (refnum out=w612:refnum<file>, error out=w621:errorcluster)  [unwired: 1 in, 1 out]
      n204 = Close File(refnum=w612, error in=w621) -> (error out=w605:errorcluster)  [unwired: 1 out]
      n205 = call-poly "IMAQ Write File 2"("error in (no error)"=w605, "Image Quality"=u32 1000, "File Path"=w607, "Image"=w606) -> ("error out"=w604:errorcluster)  [unwired: 6 in, 1 out]
    }
  }
  "error out" <- w79
